vi "ep_Amplitude and Phase Spectrum.vi"(7 "# of bins":u16, 8 "error in (no error)":errorcluster, 11 "waveform":waveform(dbl)) -> (0 "error out":errorcluster, 3 "spectrum":T2)   [LabVIEW 2013, in "NI_EP_Power Quality.lvlib"]
uses:
  <vilib>/addons/Electrical Power/PQ/NI_EP_Power Quality.lvlib
  <vilib>/addons/Electrical Power/PQ/Common/Controls/ep_AI Data Channel.ctl
  <vilib>/addons/Electrical Power/Power Measurement/NI_EP_Power Measurement.lvlib
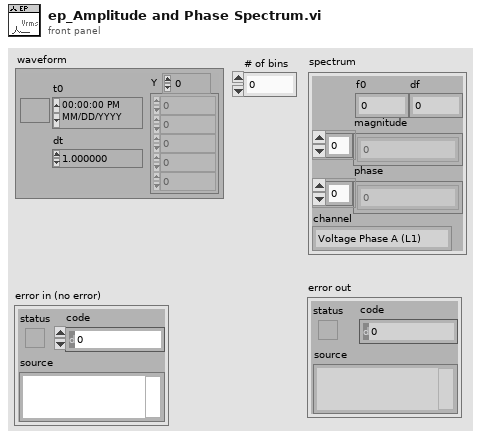
[diagram p1: front panel]
types:
  T1 = typedef "NI_EP_Power Quality.lvlib/ep_AI Data Channel.ctl" = enum16{"Voltage Phase A (L1)", "Voltage Phase B (L2)", "Voltage Phase C (L3)", "Voltage Phase N (Neutral)", "Current Phase A (L1)", "Current Phase B (L2)", "Current Phase C (L3)", "Current Phase N (Neutral)"}
  T2 = cluster{"f0":dbl, "df":dbl, "magnitude":dbl[], "phase":dbl[], "channel":T1}
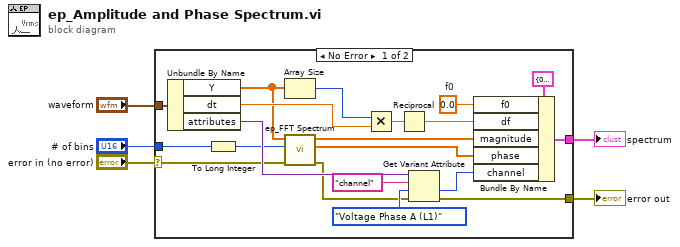
[diagram p0: block diagram]
diagram:
  n1 = case shown="No Error" "error in (no error)" {
    selector: "error in (no error)" -> [w6 w26]
    tunnel: "# of bins" -> [w23 _]
    tunnel: "waveform" -> [w20 _]
    tunnel: [w14 w26] -> w3
    tunnel: [w10 _] -> w2
    frame No Error {
      w22 = 0.0  # f0
      n2 = Unbundle By Name(w20) -> ("Y"=w13:dbl[], "dt"=w19:dbl, "attributes"=w16:variant)
      n3 = To Long Integer(number=w23) -> (32bit integer=w12:i32)
      n4 = Array Size(array=w13) -> (size(s)=w24:i32)
      n5 = call <vilib>:"ep_FFT Spectrum.vi"("error in (no error)"=w6, "# of bins"=w12, "resampled signal"=w13) -> ("error out"=w11:errorcluster, "phase"=w7:dbl[], "magnitude"=w8:dbl[])  [unwired: 6 in]
      n6 = Multiply(x=w24, y=w19) -> (x*y=w25:dbl)
      n7 = Reciprocal(x=w25) -> (1/x=w21:dbl)
      n8 = Get Variant Attribute(Variant=w16, name="channel", default value (empty Variant)=ep_AI_Data_Channel."Voltage Phase A (L1)" ("AI data channel"), error in=w11) -> (value=w15:T1, error out=w14:errorcluster)  [unwired: 2 out]
      n9 = Bundle By Name(cluster=T2 {"f0"=0.0, "df"=0.0, "magnitude"=[], "phase"=[], "channel"=enum."Voltage Phase A (L1)"} ("spectrum"), "f0"=w22, "df"=w21, "magnitude"=w8, "phase"=w7, "channel"=w15) -> (w10:T2)
    }
    frame Error {
    }
  }
  "spectrum" <- w2
  "error out" <- w3
